vi "Bind.vi"(8 "error in":errorcluster, 10 "endpoint":string="tcp://", 11 "socket in":refnum<class "Socket.lvclass">) -> (0 "error out":errorcluster, 3 "socket out":refnum<class "Socket.lvclass">)   [LabVIEW 2025, in "ZeroMQ.lvlib" / "Socket.lvclass"]
doc: "Bind a socket to a particular <b>endpoint</b>. This is somewhat similiar to \"listening\" for a connection.\n\nThe endpoint string specifies the protocol and the port to accept connection from. In this instance the originating host and port may each be wildcarded (*).\n\nExamples for \"endpoint\":\n tcp://localhost:1234\n tcp://*:5432\n inproc://namedprocess\n\nDetailed API documentation: http://api.zeromq.org/3-2:zmq-bind"
uses:
  Socket.lvclass
  Socket.lvclass/Socket.ctl
  libzmq-v143-mt-4_3_6/LibZMQ.lvlib
panel:
  # "ØMQ"
  # "labview"
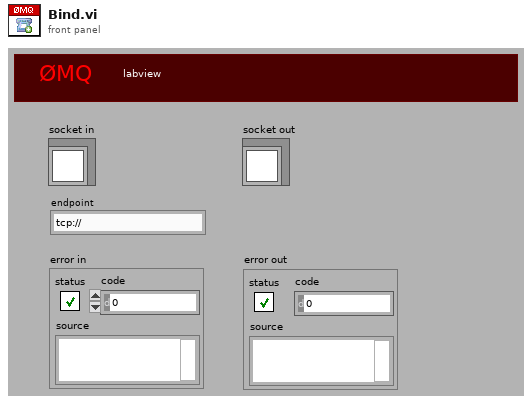
[diagram p1: front panel]
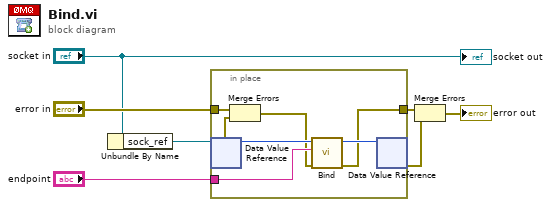
[diagram p0: block diagram]
diagram:
  n1 = Unbundle By Name("socket in") -> ("sock_ref"=w3:refnum<data-value>)
  n2 = in-place {
    in-place-border: "endpoint" -> [w10]
    in-place-border: "error in" -> [w14]
    in-place-border: [w8] -> w5
    n3 = in-place-dvr #1(w3) -> (w12:u64, w13:errorcluster)
    n4 = Merge Errors(w14, w13) -> (w9:errorcluster)
    n5 = call "Bind.vi"("error in (no error)"=w9, "addr_"=w10, "s_"=w12) -> ("error out"=w8:errorcluster, "s_ out"=w11:u64)  [unwired: 7 in]
    n6 = in-place-dvr #1(w11) -> (w1:errorcluster)  [unwired: 1 out]
  }
  n7 = Merge Errors(w5, w1) -> (→"error out":errorcluster)
  "socket out" <- "socket in"
